vi "ReadPyro.vi"(11 "Path":path) -> (0 "Y":i16[](array[numeric]), 1 "X":i16[](array[numeric]), 2 "Pyro2":i16[](array[numeric]), 3 "Pyro1":i16[](array[numeric]), 4 "Length":i32)   [LabVIEW 2014]
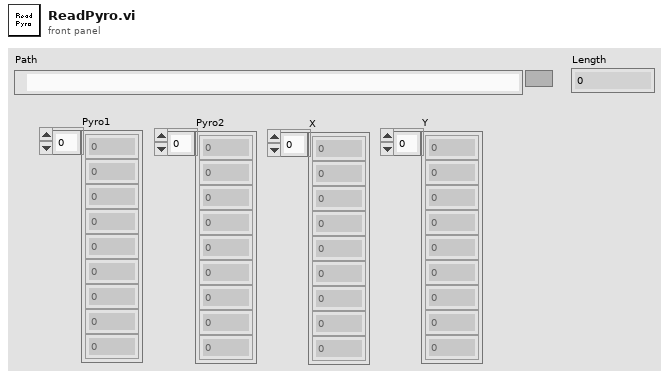
[diagram p1: front panel]
types:
  T1 = enum16{"big-endian, network order", "native, host order", "little-endian"}
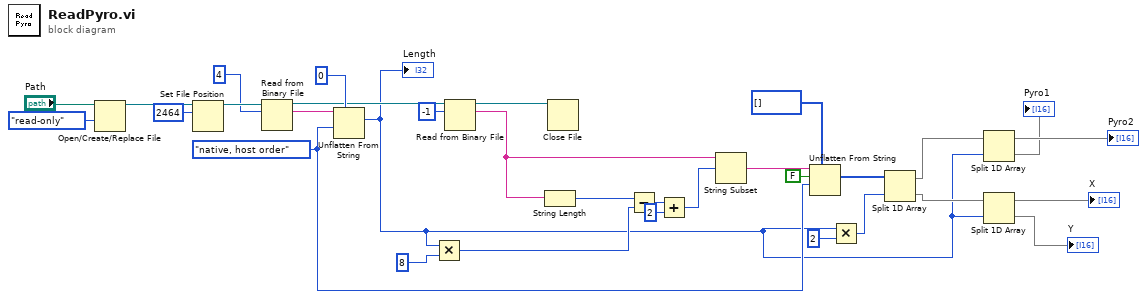
[diagram p0: block diagram]
diagram:
  w15 = T1."native, host order" ("byte order (0:big-endian, network order)")
  n1 = Open/Create/Replace File(file path (use dialog)="Path", access (0:read/write)=enum16{"read/write", "read-only", "write-only"}."read-only") -> (refnum out=w26:refnum<file>)  [unwired: 4 in, 2 out]
  n2 = Set File Position(offset (in bytes) (0)=i64 2464, refnum=w26) -> (refnum out=w30:refnum<file>)  [unwired: 2 in, 1 out]
  n3 = Read from Binary File(10:4 ("count (1)"), 11:w30) -> (2:w28:string, 3:w24:refnum<file>)  [unwired: 4 in, 2 out]
  n4 = Unflatten From String(type=0, binary string=w28, byte order (0:big-endian, network order)=w15) -> (value=w4:i32)  [unwired: 2 in, 2 out]
  "Length" <- w4
  n5 = Multiply(x=w4, y=8) -> (x*y=w19:i32)
  n6 = Read from Binary File(10:-1 ("count (1)"), 11:w24) -> (2:w18:string, 3:w23:refnum<file>)  [unwired: 4 in, 2 out]
  n7 = String Length(string=w18) -> (length=w21:i32)
  n8 = Close File(refnum=w23) -> ()  [unwired: 1 in, 2 out]
  n9 = Subtract(x=w21, y=w19) -> (x-y=w3:i32)
  n10 = Add(x=w3, y=2) -> (x+y=w2:i32)
  n11 = String Subset(string=w18, offset (0)=w2) -> (substring=w17:string)  [unwired: 1 in]
  n12 = Unflatten From String(type=i16[] [], binary string=w17, data includes array or string size? (T)=FALSE, byte order (0:big-endian, network order)=w15) -> (value=w13:i16[])  [unwired: 1 in, 2 out]
  n13 = Multiply(x=w4, y=2) -> (x*y=w11:i32)
  n14 = Split 1D Array(array=w13, index=w11) -> (first subarray=w10:i16[], second subarray=w9:i16[])
  n15 = Split 1D Array(array=w10, index=w4) -> (first subarray=→"Pyro2":i16[], second subarray=→"Pyro1":i16[])
  n16 = Split 1D Array(array=w9, index=w4) -> (first subarray=→"X":i16[], second subarray=→"Y":i16[])
